vi "Day 01 (Part Two).vi"() -> ()   [LabVIEW 2021]
panel:
  out "result":i32
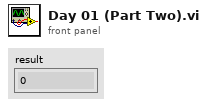
[diagram p1: front panel]
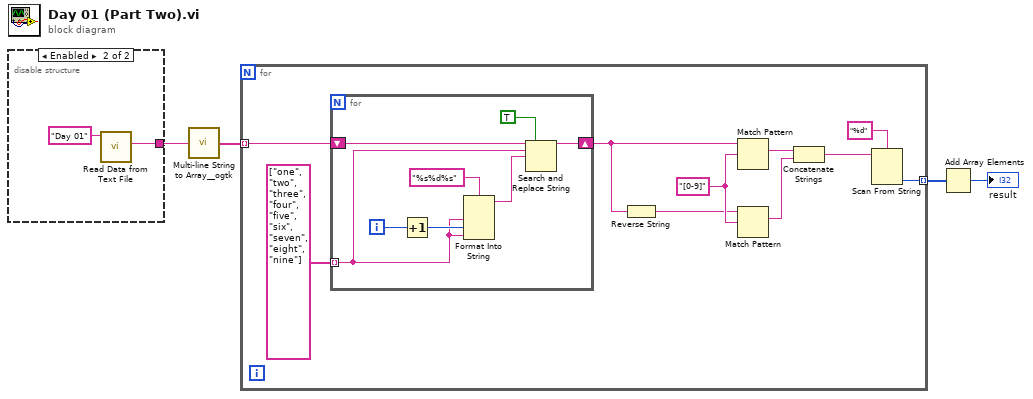
[diagram p0: block diagram]
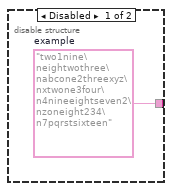
[diagram p2: hidden frame]
diagram:
  n1 = disable-structure shown="Enabled" {
    disable-tunnel: [w5 w6] -> w1
    frame Disabled {
      w5 = "two1nine\neightwothree\nabcone2threexyz\nxtwone3four\n4nineeightseven2\nzoneight234\n7pqrstsixteen"  # example
    }
    frame Enabled {
      n2 = call "Read Data from Text File.vi"("Subfolder"="Day 01") -> ("data"=w6:string)  [unwired: 10 in]
    }
  }
  n3 = call <userlib>:"Multi-line String to Array__ogtk.vi"("string"=w1) -> ("lines"=w4:string[])
  n4 = for {
    tunnel: w4 -> [w9] mode=indexing
    tunnel: [w11] -> w3 mode=indexing
    w17 = "[0-9]" ("regular expression")
    n5 = for {
      tunnel: string[] ["one", "two", "three", "four", "five", "six", "seven", "eight", "nine"] -> [w18] mode=indexing
      shift-right: [w21] -> w8
      shift-left: w9 -> [w25]
      i -> [w23]
      n6 = Increment(x=w23) -> (x+1=w19:i32)
      n7 = Format Into String(format string="%s%d%s", w18, w19, w18) -> (resulting string=w22:string)  [unwired: 2 in, 1 out]
      n8 = Search and Replace String(replace all?=TRUE ("replace all? (F)"), input string=w25, search string=w18, replace string=w22) -> (result string=w21:string)  [unwired: 4 in, 3 out]
    }
    n9 = Reverse String(1:w8) -> (0:w16:string)
    n10 = Match Pattern(string=w8, regular expression=w17) -> (match substring=w15:string)  [unwired: 1 in, 3 out]
    n11 = Match Pattern(string=w16, regular expression=w17) -> (match substring=w14:string)  [unwired: 1 in, 3 out]
    n12 = Concatenate Strings(w15, w14) -> (w12:string)
    n13 = Scan From String(format string="%d", input string=w12) -> (output 1=w11:i32)  [unwired: 3 in, 3 out]
  }
  n14 = Add Array Elements(numeric array=w3) -> (sum=→"result":i32)
